vi "String_MeasParameters_v2.vi"(11 "String":string="Measure for 0.001 seconds every 0.100 seconds, timeout 300.0 sec, 1 averages") -> (0 "averages":i16=300, 1 "timeout":dbl=300.0, 2 "rate":dbl=300.0, 3 "#seconds":dbl=300.0)   [LabVIEW 2017]
panel:
  # "Measure for 0.001 seconds every 0.100 seconds, timeout 300.0 sec, 1 averages"
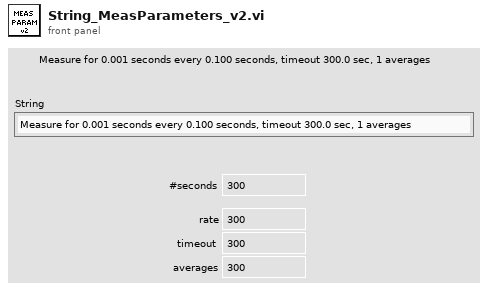
[diagram p1: front panel]
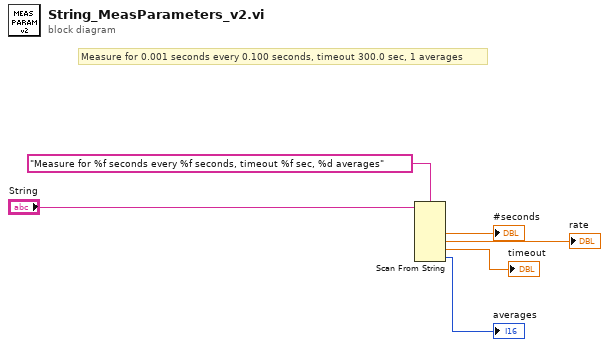
[diagram p0: block diagram]
diagram:
  # "Measure for 0.001 seconds every 0.100 seconds, timeout 300.0 sec, 1 averages"
  n1 = Scan From String(format string="Measure for %f seconds every %f seconds, timeout %f sec, %d averages", input string="String") -> (output 1=→"#seconds":dbl, output 2=→"rate":dbl, output 3=→"timeout":dbl, output 4=→"averages":i16)  [unwired: 6 in, 3 out]
